vi "SweepB_NoRecord.vi"(2 "Sweep Rate w/o recording (T/min)":dbl, 3 "Target Field (T)":dbl) -> ()   [LabVIEW 2017]
panel:
  out "Communication":string
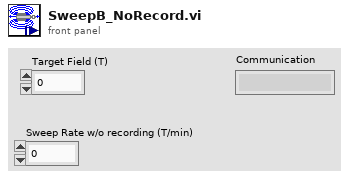
[diagram p1: front panel]
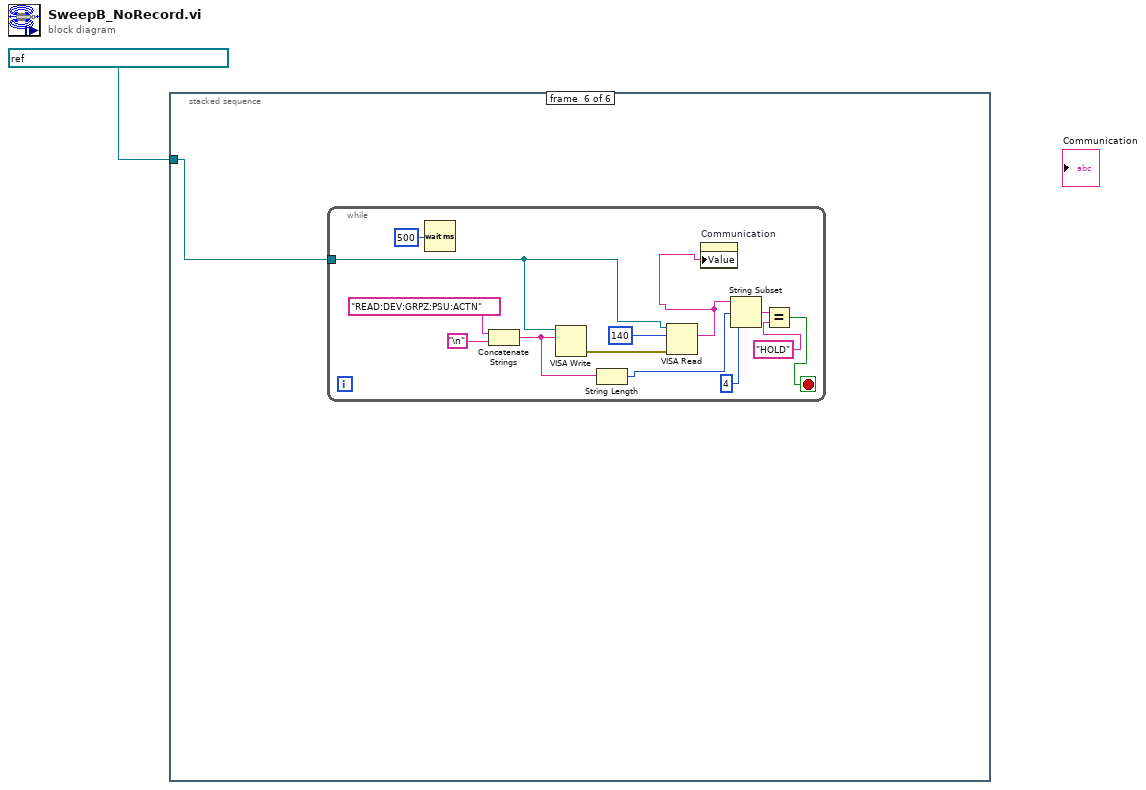
[diagram p0: block diagram]
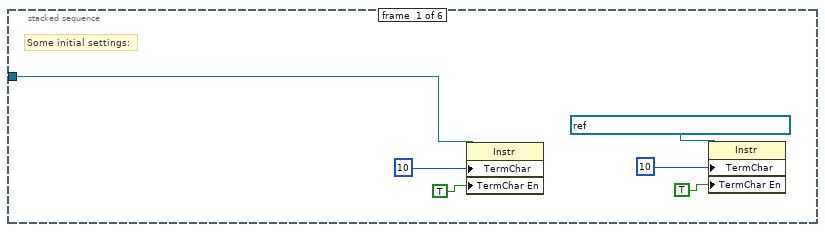
[diagram p2: hidden frame]
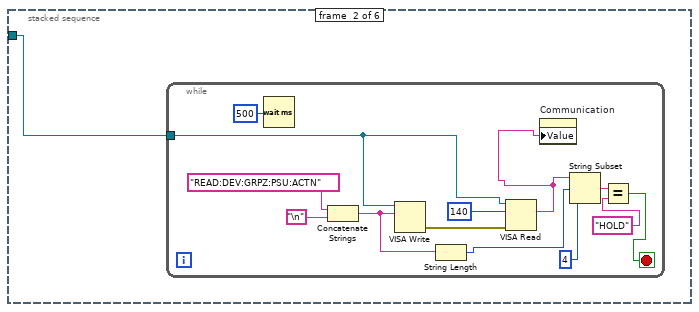
[diagram p3: hidden frame]
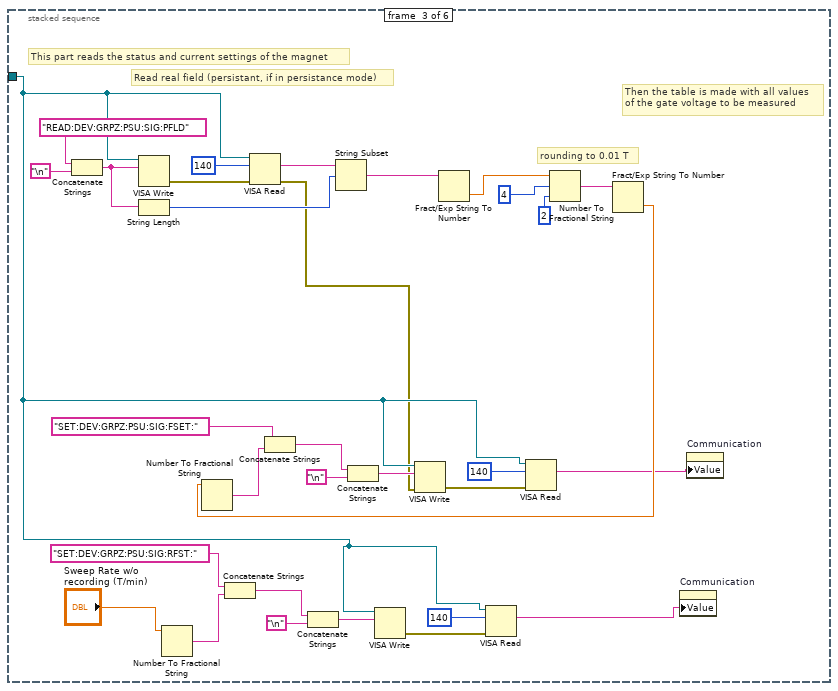
[diagram p4: hidden frame]
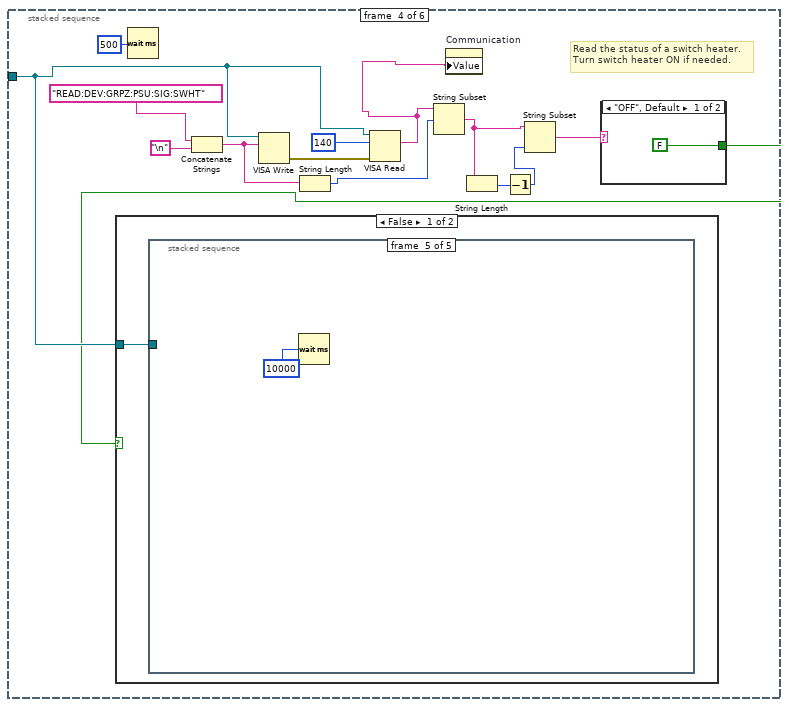
[diagram p5: hidden frame]
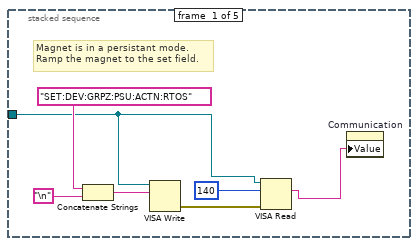
[diagram p6: hidden frame]
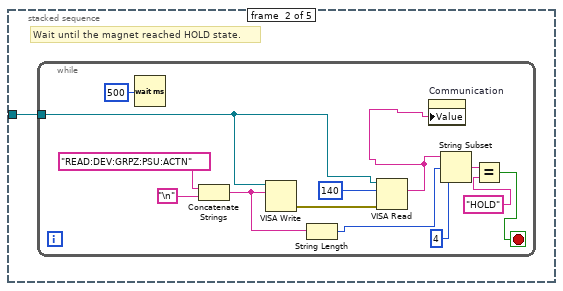
[diagram p7: hidden frame]
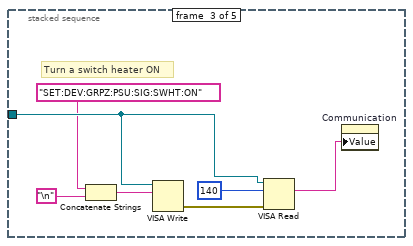
[diagram p8: hidden frame]
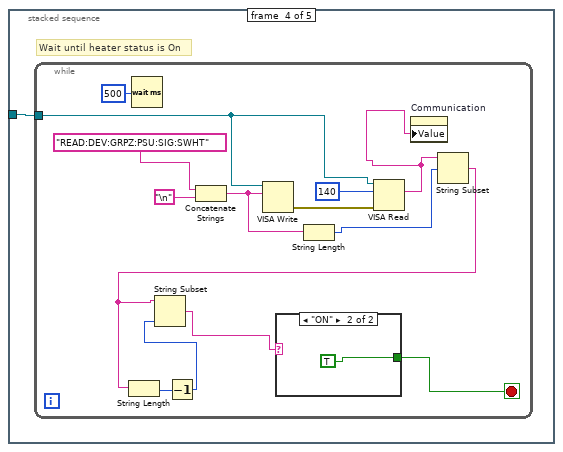
[diagram p9: hidden frame]
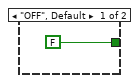
[diagram p10: hidden frame]
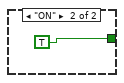
[diagram p12: hidden frame]
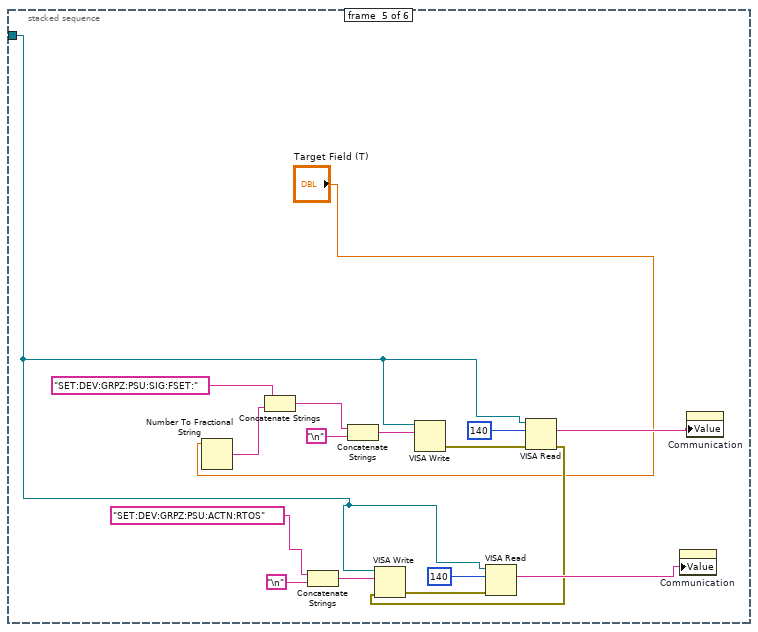
[diagram p13: hidden frame]
diagram:
  n1 = stacked-sequence {
    tunnel: refnum<visa-resource-name> "TCPIP0::192.168.128.3::7020::SOCKET" ("VISA resource name") -> [w2 w8 w25 w55 w121 w134]
    frame #0 {
      # "Some initial settings:"
      n2 = property class="Instr"(reference=w2, "TermChar"=10, "TermChar En"=TRUE) -> ()  [unwired: 1 in, 2 out]
      n3 = property class="Instr"(reference=refnum<visa-resource-name> "TCPIP0::192.168.128.2::7020::SOCKET" ("VISA resource name"), "TermChar"=10, "TermChar En"=TRUE) -> ()  [unwired: 1 in, 2 out]
    }
    frame #1 {
      n4 = while {
        tunnel: w8 -> [w18]
        stop <- w11 stop-if-true
        n5 = Wait (ms)(milliseconds to wait=500) -> ()  [unwired: 1 out]
        n6 = Concatenate Strings("READ:DEV:GRPZ:PSU:ACTN" ("string"), "\n") -> (w15:string)
        n7 = VISA Write(VISA resource name=w18, write buffer=w15) -> (error out=w21:errorcluster)  [unwired: 1 in, 2 out]
        n8 = String Length(string=w15) -> (length=w14:i32)
        n9 = VISA Read(VISA resource name=w18, byte count=140, error in (no error)=w21) -> (read buffer=w9:string)  [unwired: 3 out]
        n10 = property on="Communication" class="Str"("Value"=w9) -> ()  [unwired: 2 in, 2 out]
        n11 = String Subset(string=w9, offset (0)=w14, length (rest)=4) -> (substring=w13:string)
        n12 = Equal?(x=w13, y="HOLD") -> (x = y?=w11:bool)
      }
    }
    frame #2 {
      # "Read real field (persistant, if in persistance mode)"
      # "Then the table is made with all values\nof the gate voltage to be measured"
      # "rounding to 0.01 T"
      # "This part reads the status and current settings of the magnet"
      n13 = Concatenate Strings("READ:DEV:GRPZ:PSU:SIG:PFLD" ("string"), "\n") -> (w44:string)
      n14 = VISA Write(VISA resource name=w25, write buffer=w44) -> (error out=w50:errorcluster)  [unwired: 1 in, 2 out]
      n15 = String Length(string=w44) -> (length=w45:i32)
      n16 = Number To Fractional String(number="Sweep Rate w/o recording (T/min)") -> (F-format string=w32:string)  [unwired: 3 in]
      n17 = Concatenate Strings("SET:DEV:GRPZ:PSU:SIG:RFST:" ("string"), w32) -> (w27:string)
      n18 = VISA Read(VISA resource name=w25, byte count=140, error in (no error)=w50) -> (read buffer=w46:string, error out=w23:errorcluster)  [unwired: 2 out]
      n19 = Concatenate Strings(w27, "\n") -> (w28:string)
      n20 = String Subset(string=w46, offset (0)=w45) -> (substring=w43:string)  [unwired: 1 in]
      n21 = VISA Write(VISA resource name=w25, write buffer=w28) -> (error out=w31:errorcluster)  [unwired: 1 in, 2 out]
      n22 = Fract/Exp String To Number(string=w43) -> (number=w42:dbl)  [unwired: 3 in, 1 out]
      n23 = VISA Read(VISA resource name=w25, byte count=140, error in (no error)=w31) -> (read buffer=w24:string)  [unwired: 3 out]
      n24 = Number To Fractional String(number=w42, width (-)=4, precision (6)=2) -> (F-format string=w51:string)  [unwired: 1 in]
      n25 = Fract/Exp String To Number(string=w51) -> (number=w34:dbl)  [unwired: 3 in, 1 out]
      n26 = Number To Fractional String(number=w34) -> (F-format string=w40:string)  [unwired: 3 in]
      n27 = Concatenate Strings("SET:DEV:GRPZ:PSU:SIG:FSET:" ("string"), w40) -> (w35:string)
      n28 = Concatenate Strings(w35, "\n") -> (w36:string)
      n29 = VISA Write(VISA resource name=w25, write buffer=w36, error in (no error)=w23) -> (error out=w39:errorcluster)  [unwired: 2 out]
      n30 = VISA Read(VISA resource name=w25, byte count=140, error in (no error)=w39) -> (read buffer=w33:string)  [unwired: 3 out]
      n31 = property on="Communication" class="Str"("Value"=w24) -> ()  [unwired: 2 in, 2 out]
      n32 = property on="Communication" class="Str"("Value"=w33) -> ()  [unwired: 2 in, 2 out]
    }
    frame #3 {
      # "Read the status of a switch heater.\nTurn switch heater ON if needed."
      n33 = Wait (ms)(milliseconds to wait=500) -> ()  [unwired: 1 out]
      n34 = Concatenate Strings("READ:DEV:GRPZ:PSU:SIG:SWHT" ("string"), "\n") -> (w64:string)
      n35 = VISA Write(VISA resource name=w55, write buffer=w64) -> (error out=w67:errorcluster)  [unwired: 1 in, 2 out]
      n36 = String Length(string=w64) -> (length=w63:i32)
      n37 = VISA Read(VISA resource name=w55, byte count=140, error in (no error)=w67) -> (read buffer=w56:string)  [unwired: 3 out]
      n38 = String Subset(string=w56, offset (0)=w63) -> (substring=w57:string)  [unwired: 1 in]
      n39 = property on="Communication" class="Str"("Value"=w56) -> ()  [unwired: 2 in, 2 out]
      n40 = String Length(string=w57) -> (length=w60:i32)
      n41 = Decrement(x=w60) -> (x-1=w59:i32)
      n42 = String Subset(string=w57, length (rest)=w59) -> (substring=w58:string)  [unwired: 1 in]
      n43 = case shown="\"OFF\", Default" w58 {
        tunnel: [FALSE TRUE] -> w54
        frame "OFF", Default {
        }
        frame "ON" {
        }
      }
      n44 = case shown="False" w54 {
        tunnel: w55 -> [w68 _]
        frame False {
          n45 = stacked-sequence {
            tunnel: w68 -> [w70 w76 w92 w97 _]
            frame #0 {
              # "Magnet is in a persistant mode.\nRamp the magnet to the set field."
              n46 = Concatenate Strings("SET:DEV:GRPZ:PSU:ACTN:RTOS" ("string"), "\n") -> (w72:string)
              n47 = VISA Write(VISA resource name=w70, write buffer=w72) -> (error out=w75:errorcluster)  [unwired: 1 in, 2 out]
              n48 = VISA Read(VISA resource name=w70, byte count=140, error in (no error)=w75) -> (read buffer=w69:string)  [unwired: 3 out]
              n49 = property on="Communication" class="Str"("Value"=w69) -> ()  [unwired: 2 in, 2 out]
            }
            frame #1 {
              # "Wait until the magnet reached HOLD state."
              n50 = while {
                tunnel: w76 -> [w86]
                stop <- w79 stop-if-true
                n51 = Wait (ms)(milliseconds to wait=500) -> ()  [unwired: 1 out]
                n52 = Concatenate Strings("READ:DEV:GRPZ:PSU:ACTN" ("string"), "\n") -> (w83:string)
                n53 = VISA Write(VISA resource name=w86, write buffer=w83) -> (error out=w89:errorcluster)  [unwired: 1 in, 2 out]
                n54 = String Length(string=w83) -> (length=w82:i32)
                n55 = VISA Read(VISA resource name=w86, byte count=140, error in (no error)=w89) -> (read buffer=w77:string)  [unwired: 3 out]
                n56 = property on="Communication" class="Str"("Value"=w77) -> ()  [unwired: 2 in, 2 out]
                n57 = String Subset(string=w77, offset (0)=w82, length (rest)=4) -> (substring=w81:string)
                n58 = Equal?(x=w81, y="HOLD") -> (x = y?=w79:bool)
              }
            }
            frame #2 {
              # "Turn a switch heater ON"
              n59 = Concatenate Strings("SET:DEV:GRPZ:PSU:SIG:SWHT:ON" ("string"), "\n") -> (w93:string)
              n60 = VISA Write(VISA resource name=w92, write buffer=w93) -> (error out=w96:errorcluster)  [unwired: 1 in, 2 out]
              n61 = VISA Read(VISA resource name=w92, byte count=140, error in (no error)=w96) -> (read buffer=w90:string)  [unwired: 3 out]
              n62 = property on="Communication" class="Str"("Value"=w90) -> ()  [unwired: 2 in, 2 out]
            }
            frame #3 {
              # "Wait until heater status is On"
              n63 = while {
                tunnel: w97 -> [w108]
                stop <- w100 stop-if-true
                n64 = Wait (ms)(milliseconds to wait=500) -> ()  [unwired: 1 out]
                n65 = Concatenate Strings("READ:DEV:GRPZ:PSU:SIG:SWHT" ("string"), "\n") -> (w107:string)
                n66 = VISA Write(VISA resource name=w108, write buffer=w107) -> (error out=w111:errorcluster)  [unwired: 1 in, 2 out]
                n67 = String Length(string=w107) -> (length=w106:i32)
                n68 = VISA Read(VISA resource name=w108, byte count=140, error in (no error)=w111) -> (read buffer=w98:string)  [unwired: 3 out]
                n69 = property on="Communication" class="Str"("Value"=w98) -> ()  [unwired: 2 in, 2 out]
                n70 = String Subset(string=w98, offset (0)=w106) -> (substring=w99:string)  [unwired: 1 in]
                n71 = String Length(string=w99) -> (length=w103:i32)
                n72 = Decrement(x=w103) -> (x-1=w102:i32)
                n73 = String Subset(string=w99, length (rest)=w102) -> (substring=w101:string)  [unwired: 1 in]
                n74 = case shown="\"ON\"" w101 {
                  tunnel: [FALSE TRUE] -> w100
                  frame "OFF", Default {
                  }
                  frame "ON" {
                  }
                }
              }
            }
            frame #4 {
              n75 = Wait (ms)(milliseconds to wait=10000) -> ()  [unwired: 1 out]
            }
          }
        }
        frame True {
        }
      }
    }
    frame #4 {
      n76 = Number To Fractional String(number="Target Field (T)") -> (F-format string=w132:string)  [unwired: 3 in]
      n77 = Concatenate Strings("SET:DEV:GRPZ:PSU:SIG:FSET:" ("string"), w132) -> (w127:string)
      n78 = Concatenate Strings("SET:DEV:GRPZ:PSU:ACTN:RTOS" ("string"), "\n") -> (w122:string)
      n79 = Concatenate Strings(w127, "\n") -> (w128:string)
      n80 = VISA Write(VISA resource name=w121, write buffer=w128) -> (error out=w131:errorcluster)  [unwired: 1 in, 2 out]
      n81 = VISA Read(VISA resource name=w121, byte count=140, error in (no error)=w131) -> (read buffer=w126:string, error out=w119:errorcluster)  [unwired: 2 out]
      n82 = VISA Write(VISA resource name=w121, write buffer=w122, error in (no error)=w119) -> (error out=w125:errorcluster)  [unwired: 2 out]
      n83 = VISA Read(VISA resource name=w121, byte count=140, error in (no error)=w125) -> (read buffer=w120:string)  [unwired: 3 out]
      n84 = property on="Communication" class="Str"("Value"=w120) -> ()  [unwired: 2 in, 2 out]
      n85 = property on="Communication" class="Str"("Value"=w126) -> ()  [unwired: 2 in, 2 out]
    }
    frame #5 {
      n86 = while {
        tunnel: w134 -> [w144]
        stop <- w137 stop-if-true
        n87 = Wait (ms)(milliseconds to wait=500) -> ()  [unwired: 1 out]
        n88 = Concatenate Strings("READ:DEV:GRPZ:PSU:ACTN" ("string"), "\n") -> (w141:string)
        n89 = VISA Write(VISA resource name=w144, write buffer=w141) -> (error out=w147:errorcluster)  [unwired: 1 in, 2 out]
        n90 = String Length(string=w141) -> (length=w140:i32)
        n91 = VISA Read(VISA resource name=w144, byte count=140, error in (no error)=w147) -> (read buffer=w135:string)  [unwired: 3 out]
        n92 = property on="Communication" class="Str"("Value"=w135) -> ()  [unwired: 2 in, 2 out]
        n93 = String Subset(string=w135, offset (0)=w140, length (rest)=4) -> (substring=w139:string)
        n94 = Equal?(x=w139, y="HOLD") -> (x = y?=w137:bool)
      }
    }
  }
